vi "Support_CheckIfVIinMemory.vi"(3 "VI name":string, 5 "error in (no error)":errorcluster) -> (17 "VI is in memory?":bool, 19 "error out":errorcluster)   [LabVIEW 2009]
doc: "Checks if VI is in memory."
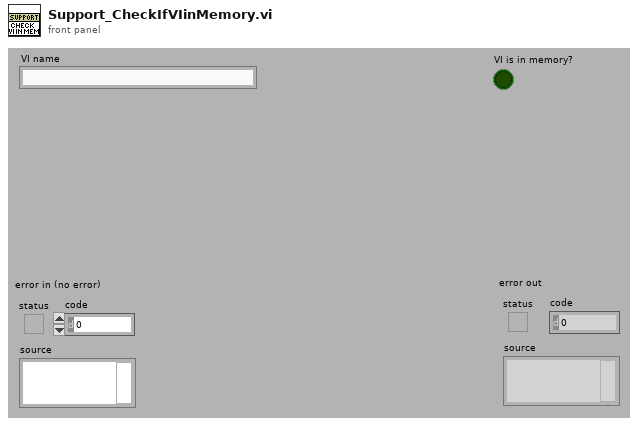
[diagram p1: front panel]
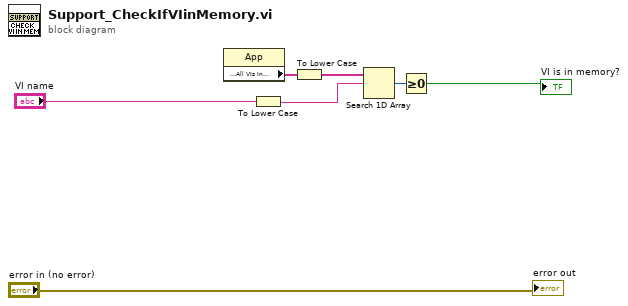
[diagram p0: block diagram]
diagram:
  n1 = property class="App"() -> ("Application:All VIs In Memory"=w6:string[])  [unwired: 2 in, 2 out]
  n2 = To Lower Case(string="VI name") -> (all lower case string=w4:string)
  n3 = To Lower Case(string=w6) -> (all lower case string=w5:string[])
  n4 = Search 1D Array(1D array=w5, element=w4) -> (index of element=w2:i32)  [unwired: 1 in]
  n5 = Greater Or Equal To 0?(x=w2) -> (x >= 0?=→"VI is in memory?":bool)
  "error out" <- "error in (no error)"
